vi "Save data.vi"(10 "Auto Data":T2(array[cluster]), 11 "File":path) -> ()   [LabVIEW 2012]
uses:
  <vilib>/Rock Robotics/WPI/Solenoid/WPI_SolenoidValue.ctl
panel:
  # "Drive Motor 1"
  # "Drive Motor 2"
  # "Scaling Value"
  # "Shooter Speed"
  # "Window Position"
  # "Shooting Solenoid"
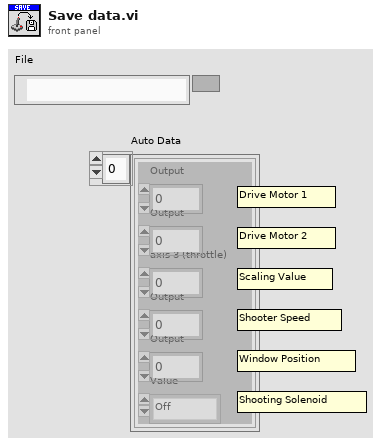
[diagram p1: front panel]
types:
  T1 = typedef "WPI_SolenoidValue.ctl" = enum16{"Off", "On", "Forward", "Reverse"}
  T2 = cluster{"Output":dbl, "Output":dbl, "axis 3 (throttle)":dbl, "Output":dbl, "Output":dbl, "Value":T1}[]
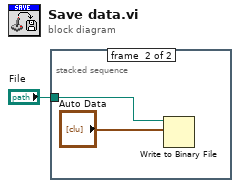
[diagram p0: block diagram]
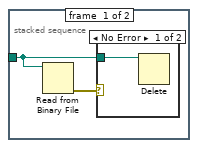
[diagram p2: hidden frame]
diagram:
  n1 = stacked-sequence {
    tunnel: "File" -> [w2 w6]
    frame #0 {
      n2 = Read from Binary File(11:w2) -> (0:w3:errorcluster)  [unwired: 5 in, 3 out]
      n3 = case shown="No Error" w3 {
        tunnel: w2 -> [w4 _]
        frame No Error {
          n4 = Delete(path (use dialog)=w4) -> ()  [unwired: 4 in, 3 out]
        }
        frame Error {
        }
      }
    }
    frame #1 {
      n5 = Write to Binary File(file (use dialog)=w6, data="Auto Data") -> ()  [unwired: 4 in, 3 out]
    }
  }
